vi "IDD.vi"(8 "error in (no error)":errorcluster, 10 "Multimetru":refnum<visa-resource-name>="GPIB0::24::INSTR", 11 "SMU":refnum<visa-resource-name>="GPIB0::1::INSTR") -> (0 "error out":errorcluster, 3 "IDD":dbl)   [LabVIEW 2020]
uses:
  217e2a43-9340-4c5b-831b-a9f31957e4b5.vi
  fe0ccdfc-09ea-4e28-b1fe-2a94c257dca7.vi
  ff1688d8-c357-4d8a-9c4d-56d50204c198.vi
  8e54136d-94e3-4361-8160-c133b6c1b66a.vi
  Drivers/agilent_3446x_series/Agilent 3446X Series/Public/Data/Read (Single Point).vi
  Drivers/keithley_2450/Keithley 2450/Keithley 2450.lvlib
  Drivers/agilent_3446x_series/Agilent 3446X Series/Agilent 3446X Series.lvlib
panel:
  out "noOfDevs out":u32=1
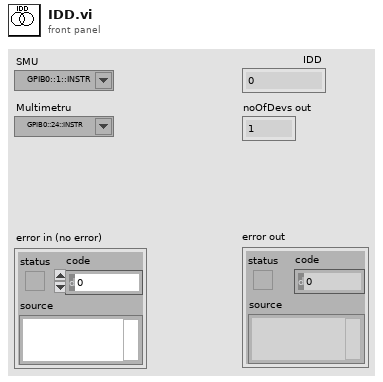
[diagram p1: front panel]
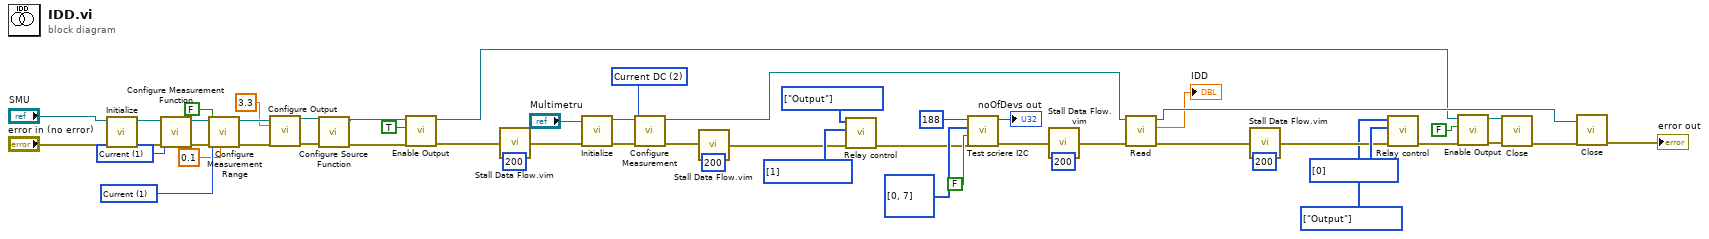
[diagram p0: block diagram]
diagram:
  w10 = u16[] [1] items=["low"=0, "high"=1, "Unchange"=255] ("outputValues")
  w11 = enum8{"Output", "Input", "Unchange"}[] [enum."Output"] items=["Output", "Input", "Unchange"] ("gpioDir")
  w23 = u16 1 items=["Volts", "Current", "Resistance"] ("Function (0: Volts)")
  w24 = u16 1 items=["Volts", "Current", "Auto Resistance", "Manual Resistance", "Digitize Voltage", "Digitize Current"] ("Function (0: Volts)")
  w31 = enum8{"Output", "Input", "Unchange"}[] [enum."Output"] items=["Output", "Input", "Unchange"] ("gpioDir")
  w33 = u16[] [0] items=["low"=0, "high"=1, "Unchange"=255] ("outputValues")
  w42 = 2 items=["Continuity", "Current AC", "Current DC", "Diode", "Frequency", "Resistance 4-wire", "Period", "Resistance 2-wire", "Temperature", "Voltage AC", "Voltage DC", "Voltage DC Ratio", "Capacitance"] ("Measurement Function (10: Voltage DC)")
  n1 = call "Initialize.vi"("error in (no error)"="error in (no error)", "VISA resource name"="SMU") -> ("error out"=w28:errorcluster, "VISA resource name out"=w29:refnum<visa-resource-name>)  [unwired: 8 in]
  n2 = call "Configure Measurement Function.vi"("error in (no error)"=w28, "Function (0: Volts)"=w24, "VISA resource name"=w29) -> ("error out"=w26:errorcluster, "VISA resource name out"=w27:refnum<visa-resource-name>)  [unwired: 7 in]
  n3 = call "Configure Measurement Range.vi"("Manual Range (1.0)"=0.1, "error in (no error)"=w26, "Enable Auto Range (T:Enable)"=FALSE, "Function (0: Volts)"=w23, "VISA resource name"=w27) -> ("error out"=w21:errorcluster, "VISA resource name out"=w22:refnum<visa-resource-name>)  [unwired: 5 in]
  n4 = call "Configure Output.vi"("VISA resource name"=w22, "Source Level (0)"=3.3, "error in (no error)"=w21) -> ("VISA resource name out"=w19:refnum<visa-resource-name>, "error out"=w18:errorcluster)  [unwired: 11 in]
  n5 = call "Configure Source Function.vi"("error in (no error)"=w18, "VISA resource name"=w19) -> ("error out"=w17:errorcluster, "VISA resource name out"=w16:refnum<visa-resource-name>)  [unwired: 8 in]
  n6 = call "Enable Output.vi"("error in (no error)"=w17, "Enable Output (T: Enable)"=TRUE, "VISA resource name"=w16) -> ("error out"=w13:errorcluster, "VISA resource name out"=w14:refnum<visa-resource-name>)  [unwired: 7 in]
  n7 = call "Stall Data Flow.vim"("value in"=w13, "milliseconds to wait"=u32 200) -> ("value out"=w35:errorcluster)  [unwired: 1 out]
  n8 = call "Initialize.vi"("error in (no error)"=w35, "VISA resource name"="Multimetru") -> ("error out"=w44:errorcluster, "VISA resource name out"=w43:refnum<visa-resource-name>)  [unwired: 8 in]
  n9 = call "Configure Measurement.vi"("error in (no error)"=w44, "Measurement Function (10: Voltage DC)"=w42, "VISA resource name"=w43) -> ("error out"=w9:errorcluster, "VISA resource name out"=w8:refnum<visa-resource-name>)  [unwired: 7 in]
  n10 = call "Stall Data Flow.vim"("value in"=w9, "milliseconds to wait"=u32 200) -> ("value out"=w2:errorcluster)  [unwired: 1 out]
  n11 = call "Relay control.vi"("error in (no error) 2"=w2, "outputValues"=w10, "gpioDir"=w11) -> ("error out"=w1:errorcluster)  [unwired: 8 in]
  n12 = call "Test scriere I2C.vi"("error in (no error)"=w1, "use7bitAddress"=FALSE, "i2cTxData"=u8[] [0, 7], "slaveAddress"=u8 188) -> ("error out"=w3:errorcluster, "noOfDevs out"=→"noOfDevs out":u32)  [unwired: 5 in, 1 out]
  n13 = call "Stall Data Flow.vim"("value in"=w3, "milliseconds to wait"=u32 200) -> ("value out"=w40:errorcluster)  [unwired: 1 out]
  n14 = call-poly "Read.vi"("error in (no error)"=w40, "VISA resource name"=w8) -> ("error out"=w37:errorcluster, "Measurement"=→"IDD":dbl, "VISA resource name out"=w39:refnum<visa-resource-name>)  [unwired: 7 in]
  n15 = call "Stall Data Flow.vim"("value in"=w37, "milliseconds to wait"=u32 200) -> ("value out"=w32:errorcluster)  [unwired: 1 out]
  n16 = call "Relay control.vi"("error in (no error) 2"=w32, "outputValues"=w33, "gpioDir"=w31) -> ("error out"=w30:errorcluster)  [unwired: 8 in]
  n17 = call "Enable Output.vi"("error in (no error)"=w30, "Enable Output (T: Enable)"=FALSE, "VISA resource name"=w14) -> ("error out"=w48:errorcluster, "VISA resource name out"=w49:refnum<visa-resource-name>)  [unwired: 7 in]
  n18 = call "Close.vi"("error in (no error)"=w48, "VISA resource name"=w49) -> ("error out"=w46:errorcluster)  [unwired: 9 in]
  n19 = call "Close.vi"("error in (no error)"=w46, "VISA resource name"=w39) -> ("error out"=→"error out":errorcluster)  [unwired: 9 in]
